vi "Set Voltage.vi"(8 "error in (no error)":errorcluster, 10 "Voltage":dbl, 11 "PS_Sim in":refnum<class "PS Simulated.lvclass">) -> (0 "error out":errorcluster, 3 "PS_Sim out":refnum<class "PS Simulated.lvclass">)   [LabVIEW 2021, in "PS.lvlib" / "PS Simulated.lvclass"]
uses:
  PS Simulated.lvclass
  PS Simulated.lvclass/PS Simulated.ctl
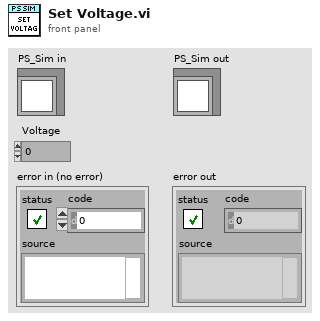
[diagram p1: front panel]
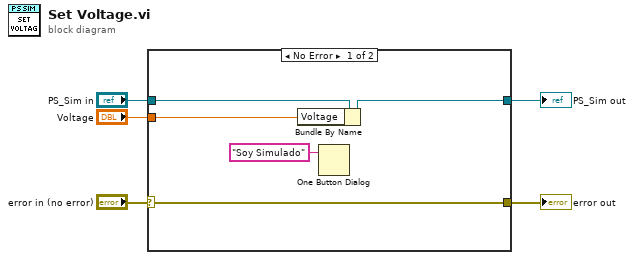
[diagram p0: block diagram]
diagram:
  n1 = case shown="No Error" "error in (no error)" {
    selector: "error in (no error)" -> [w9 w11]
    tunnel: [w8 w12] -> w4
    tunnel: "PS_Sim in" -> [w10 w12]
    tunnel: [w9 w11] -> w2
    tunnel: "Voltage" -> [w7 _]
    frame No Error {
      n2 = Bundle By Name(cluster=w10, "Voltage"=w7) -> (w8:refnum<class "PS Simulated.lvclass">)
      n3 = One Button Dialog(message="Soy Simulado") -> ()  [unwired: 1 in, 1 out]
    }
    frame Error {
    }
  }
  "error out" <- w2
  "PS_Sim out" <- w4
